vi "GetString.vi"(7 "key description":string, 8 "sections":string[](array[string]), 9 "string":string, 11 "info data":string) -> (0 "sections out":string[](array[string]), 1 "found?":bool, 2 "value":string, 3 "info data out":string)   [LabVIEW 2013, in "infolib.lvlib"]
doc: "Add a new numeric key to Info Data string. If section exists in Info Data string, inserts key into this section."
uses:
  infolib.lvlib
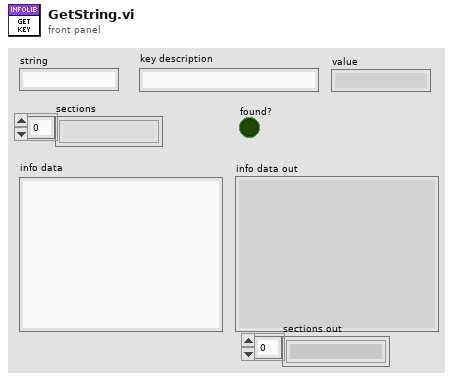
[diagram p1: front panel]
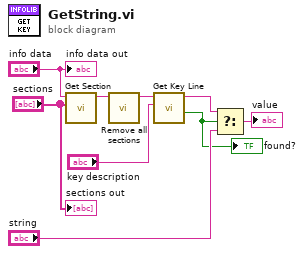
[diagram p0: block diagram]
diagram:
  n1 = call "Get Section.vi"("sections"="sections", "info data"="info data") -> ("section part"=w9:string)  [unwired: 8 in, 1 out]
  n2 = call "Remove all sections.vi"("info data"=w9) -> ("info data out"=w7:string)  [unwired: 10 in]
  n3 = call "Get Key Line.vi"("key description"="key description", "info data"=w7) -> ("key found?"=w1:bool, "key value"=w4:string)  [unwired: 7 in, 1 out]
  "found?" <- w1
  n4 = Select(t=w4, s=w1, f="string") -> (s? t:f=→"value":string)
  "info data out" <- "info data"
  "sections out" <- "sections"
